vi "IT8512AControl.vi"(8 "功能":T1(ring), 9 "输入":dbl, 10 "端口":string="INP 0") -> (1 "输出":dbl)   [LabVIEW 2018]
uses:
  <vilib>/Instr/_visa.llb/VISA Configure Serial Port (Instr).vi
panel:
  in  "error in (no error)":errorcluster caption="错误输入（无错误）"
  out "error out":errorcluster
  # "IT8512 CONTROL"
  # "r"
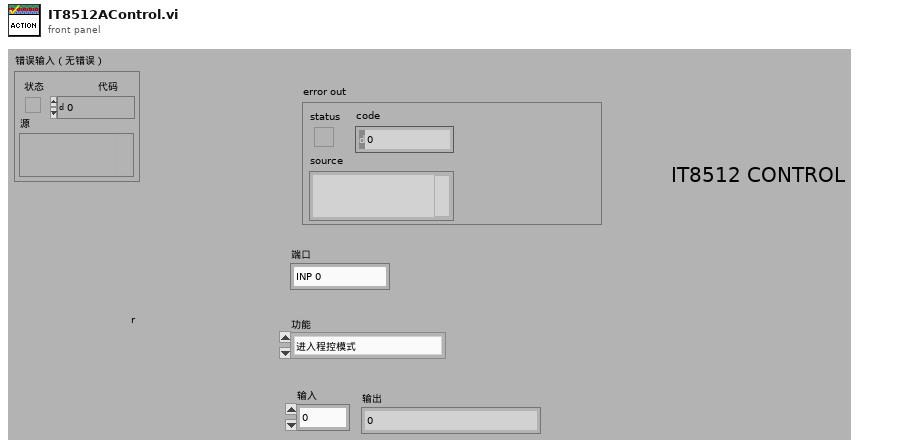
[diagram p1: front panel]
types:
  T1 = enum16{"进入程控模式", "输出ON", "输出OFF", "设置电压", "设置电流", "读取电压", "读取电流", "CC", "CV", "进入手动模式"}
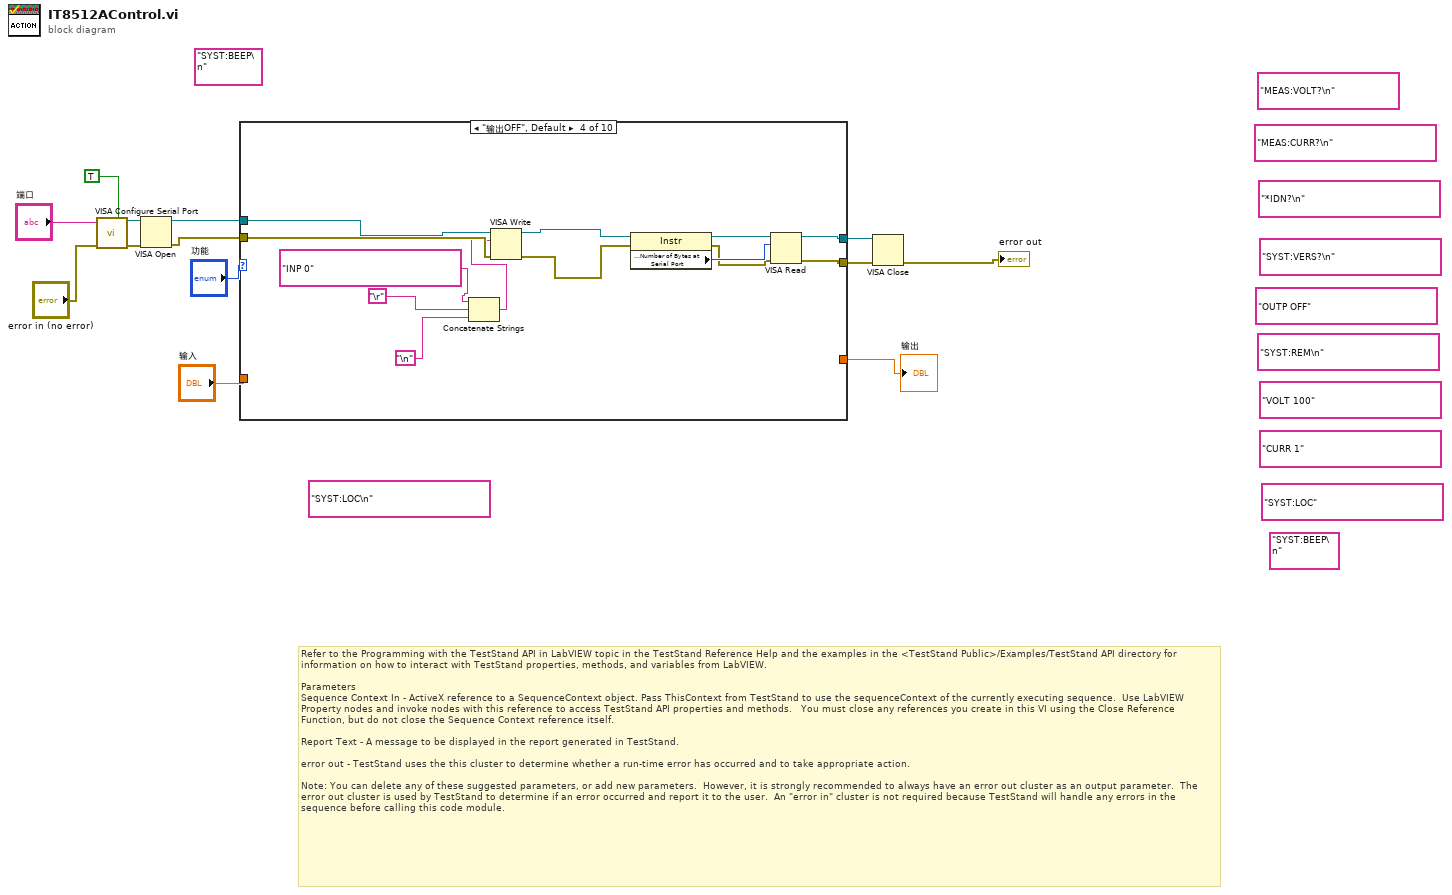
[diagram p0: block diagram]
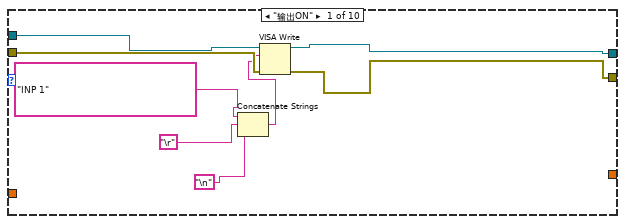
[diagram p2: hidden frame]
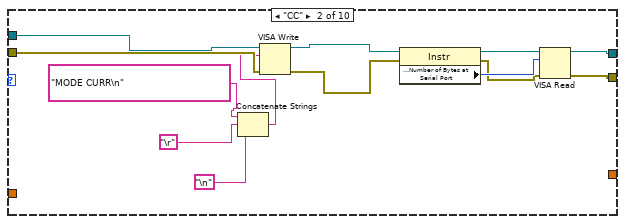
[diagram p3: hidden frame]
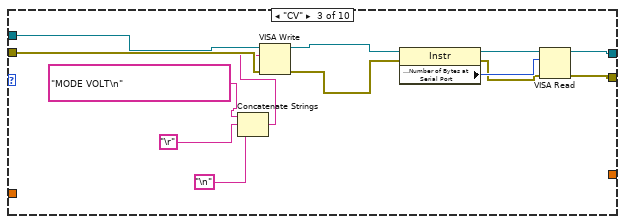
[diagram p4: hidden frame]
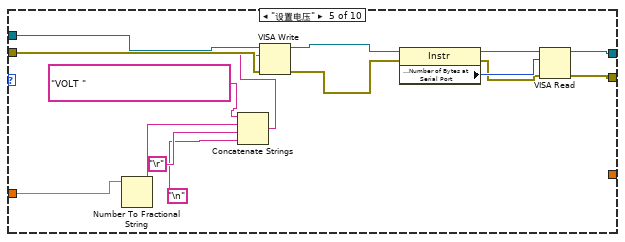
[diagram p5: hidden frame]
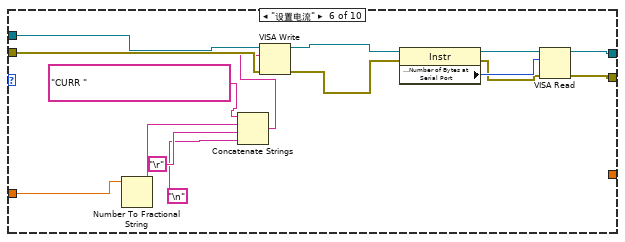
[diagram p6: hidden frame]
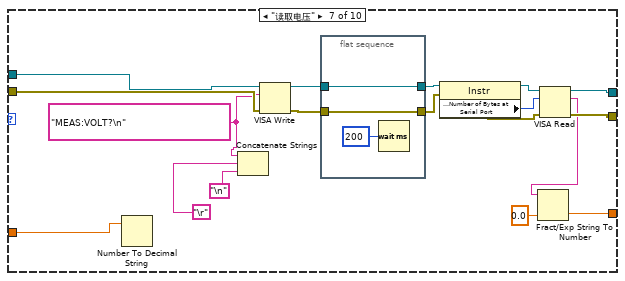
[diagram p7: hidden frame]
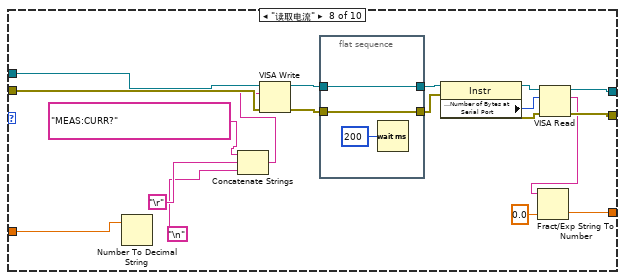
[diagram p8: hidden frame]
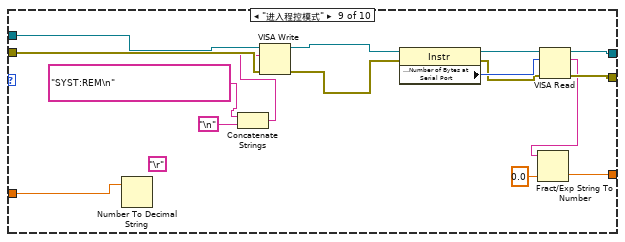
[diagram p9: hidden frame]
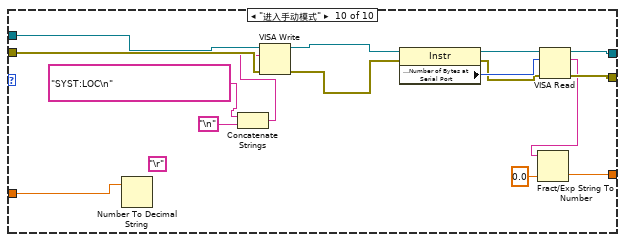
[diagram p10: hidden frame]
diagram:
  (unwired) "SYST:LOC\n" ("写入缓冲区")
  (unwired) "SYST:LOC" ("写入缓冲区")
  (unwired) "CURR 1" ("写入缓冲区")
  (unwired) "VOLT 100" ("写入缓冲区")
  (unwired) "OUTP OFF" ("写入缓冲区")
  (unwired) "SYST:REM\n" ("写入缓冲区")
  (unwired) "SYST:VERS?\n" ("写入缓冲区")
  (unwired) "*IDN?\n" ("写入缓冲区")
  (unwired) "MEAS:CURR?\n" ("写入缓冲区")
  (unwired) "MEAS:VOLT?\n" ("写入缓冲区")
  (unwired) "SYST:BEEP\n" ("写入缓冲区")
  (unwired) "SYST:BEEP\n" ("写入缓冲区")
  # "Refer to the Programming with the TestStand API in LabVIEW topic in the TestStand Reference Help and the examples in the <TestStand Public>/Examples/TestStand API directory for information on how to interact with TestStand properties, methods, and variables from LabVIEW.\n\nParameters\nSequence Context In - ActiveX reference to a SequenceContext object. Pass ThisContext from TestStand to use the sequenceContext of the currently executing sequence.  Use LabVIEW Property nodes and invoke nodes with this reference to access TestStand API properties and methods.   You must close any references you create in this VI using the Close Reference Function, but do not close the Sequence Context reference itself.\n\nReport Text - A message to be displayed in the report generated in TestStand. \n\nerror out - TestStand uses the this cluster to determine whether a run-time error has occurred and to take appropriate action.  \n\nNote: You can delete any of these suggested parameters, or add new parameters.  However, it is strongly recommended to always have an error out cluster as an output parameter.  The error out cluster is used by TestStand to determine if an error occurred and report it to the user.  An \"error in\" cluster is not required because TestStand will handle any errors in the sequence before calling this code module."
  n1 = call-poly "VISA Configure Serial Port"("VISA resource name"="端口", "Enable Termination\nChar (T)"=TRUE ("Enable Termination\nChar (T)"), "error in (no error)"="error in (no error)") -> ("VISA resource name out"=w12:refnum<visa-resource-name>, "error out"=w13:errorcluster)  [unwired: 11 in]
  n2 = VISA Open(error in (no error)=w13, VISA resource name=w12) -> (VISA resource name=w11:refnum<visa-resource-name>, error out=w10:errorcluster)  [unwired: 3 in]
  n3 = case shown="\"输出OFF\", Default" "功能" {
    tunnel: w11 -> [w21 w34 w47 w60 w75 w90 w108 w130 w149 w165]
    tunnel: w10 -> [w20 w33 w46 w59 w74 w89 w107 w129 w148 w164]
    tunnel: [w17 w27 w40 w51 w66 w81 w102 w122 w141 w157] -> w8
    tunnel: [w16 w26 w39 w50 w65 w80 w101 w121 w140 w156] -> w7
    tunnel: "输入" -> [_ _ _ _ w61 w76 w99 w119 w137 w153]
    tunnel: [_ _ _ _ _ _ w96 w116 w134 w150] -> w3
    frame "输出ON" {
      n4 = Concatenate Strings("INP 1" ("写入缓冲区"), "\r", "\n") -> (w14:string)
      n5 = VISA Write(VISA resource name=w21, write buffer=w14, error in (no error)=w20) -> (VISA resource name out=w17:refnum<visa-resource-name>, error out=w16:errorcluster)  [unwired: 1 out]
    }
    frame "CC" {
      n6 = Concatenate Strings("MODE CURR\n" ("写入缓冲区"), "\r", "\n") -> (w28:string)
      n7 = VISA Write(VISA resource name=w34, write buffer=w28, error in (no error)=w33) -> (VISA resource name out=w32:refnum<visa-resource-name>, error out=w24:errorcluster)  [unwired: 1 out]
      n8 = property class="Instr"(reference=w32, error in=w24) -> (reference out=w31:refnum<visa-resource-name>, error out=w25:errorcluster, "Serial Settings:Number of Bytes at Serial Port"=w30:u32)
      n9 = VISA Read(VISA resource name=w31, byte count=w30, error in (no error)=w25) -> (VISA resource name out=w27:refnum<visa-resource-name>, error out=w26:errorcluster)  [unwired: 2 out]
    }
    frame "CV" {
      n10 = Concatenate Strings("MODE VOLT\n" ("写入缓冲区"), "\r", "\n") -> (w41:string)
      n11 = VISA Write(VISA resource name=w47, write buffer=w41, error in (no error)=w46) -> (VISA resource name out=w45:refnum<visa-resource-name>, error out=w37:errorcluster)  [unwired: 1 out]
      n12 = property class="Instr"(reference=w45, error in=w37) -> (reference out=w44:refnum<visa-resource-name>, error out=w38:errorcluster, "Serial Settings:Number of Bytes at Serial Port"=w43:u32)
      n13 = VISA Read(VISA resource name=w44, byte count=w43, error in (no error)=w38) -> (VISA resource name out=w40:refnum<visa-resource-name>, error out=w39:errorcluster)  [unwired: 2 out]
    }
    frame "输出OFF", Default {
      n14 = Concatenate Strings("INP 0" ("写入缓冲区"), "\r", "\n") -> (w54:string)
      n15 = VISA Write(VISA resource name=w60, write buffer=w54, error in (no error)=w59) -> (VISA resource name out=w58:refnum<visa-resource-name>, error out=w48:errorcluster)  [unwired: 1 out]
      n16 = property class="Instr"(reference=w58, error in=w48) -> (reference out=w57:refnum<visa-resource-name>, error out=w49:errorcluster, "Serial Settings:Number of Bytes at Serial Port"=w56:u32)
      n17 = VISA Read(VISA resource name=w57, byte count=w56, error in (no error)=w49) -> (VISA resource name out=w51:refnum<visa-resource-name>, error out=w50:errorcluster)  [unwired: 2 out]
    }
    frame "设置电压" {
      n18 = Number To Fractional String(number=w61) -> (F-format string=w62:string)  [unwired: 3 in]
      n19 = Concatenate Strings("VOLT " ("写入缓冲区"), w62, "\r", "\n") -> (w69:string)
      n20 = VISA Write(VISA resource name=w75, write buffer=w69, error in (no error)=w74) -> (VISA resource name out=w73:refnum<visa-resource-name>, error out=w63:errorcluster)  [unwired: 1 out]
      n21 = property class="Instr"(reference=w73, error in=w63) -> (reference out=w72:refnum<visa-resource-name>, error out=w64:errorcluster, "Serial Settings:Number of Bytes at Serial Port"=w71:u32)
      n22 = VISA Read(VISA resource name=w72, byte count=w71, error in (no error)=w64) -> (VISA resource name out=w66:refnum<visa-resource-name>, error out=w65:errorcluster)  [unwired: 2 out]
    }
    frame "设置电流" {
      n23 = Number To Fractional String(number=w76) -> (F-format string=w77:string)  [unwired: 3 in]
      n24 = Concatenate Strings("CURR " ("写入缓冲区"), w77, "\r", "\n") -> (w84:string)
      n25 = VISA Write(VISA resource name=w90, write buffer=w84, error in (no error)=w89) -> (VISA resource name out=w88:refnum<visa-resource-name>, error out=w78:errorcluster)  [unwired: 1 out]
      n26 = property class="Instr"(reference=w88, error in=w78) -> (reference out=w87:refnum<visa-resource-name>, error out=w79:errorcluster, "Serial Settings:Number of Bytes at Serial Port"=w86:u32)
      n27 = VISA Read(VISA resource name=w87, byte count=w86, error in (no error)=w79) -> (VISA resource name out=w81:refnum<visa-resource-name>, error out=w80:errorcluster)  [unwired: 2 out]
    }
    frame "读取电压" {
      w95 = "MEAS:VOLT?\n" ("写入缓冲区")
      n28 = Number To Decimal String(number=w99) -> ()  [unwired: 1 in, 1 out]
      n29 = Concatenate Strings(w95, "\r", "\n") -> ()  [unwired: 1 out]
      n30 = VISA Write(VISA resource name=w108, write buffer=w95, error in (no error)=w107) -> (VISA resource name out=w93:refnum<visa-resource-name>, error out=w92:errorcluster)  [unwired: 1 out]
      n31 = flat-sequence {
        tunnel: [w111] -> w94
        tunnel: w93 -> [w111]
        tunnel: w92 -> [w110]
        tunnel: [w110] -> w91
        frame #0 {
          n32 = Wait (ms)(milliseconds to wait=u32 200) -> ()  [unwired: 1 out]
        }
      }
      n33 = property class="Instr"(reference=w94, error in=w91) -> (reference out=w106:refnum<visa-resource-name>, error out=w100:errorcluster, "Serial Settings:Number of Bytes at Serial Port"=w105:u32)
      n34 = VISA Read(VISA resource name=w106, byte count=w105, error in (no error)=w100) -> (VISA resource name out=w102:refnum<visa-resource-name>, read buffer=w98:string, error out=w101:errorcluster)  [unwired: 1 out]
      n35 = Fract/Exp String To Number(string=w98, default (0 dbl)=0.0 ("默认(0 I32)")) -> (number=w96:dbl)  [unwired: 2 in, 1 out]
    }
    frame "读取电流" {
      n36 = Number To Decimal String(number=w119) -> ()  [unwired: 1 in, 1 out]
      n37 = Concatenate Strings("MEAS:CURR?" ("写入缓冲区"), "\r", "\n") -> (w125:string)
      n38 = VISA Write(VISA resource name=w130, write buffer=w125, error in (no error)=w129) -> (VISA resource name out=w115:refnum<visa-resource-name>, error out=w114:errorcluster)  [unwired: 1 out]
      n39 = flat-sequence {
        tunnel: [w133] -> w113
        tunnel: w115 -> [w133]
        tunnel: w114 -> [w132]
        tunnel: [w132] -> w112
        frame #0 {
          n40 = Wait (ms)(milliseconds to wait=u32 200) -> ()  [unwired: 1 out]
        }
      }
      n41 = property class="Instr"(reference=w113, error in=w112) -> (reference out=w128:refnum<visa-resource-name>, error out=w120:errorcluster, "Serial Settings:Number of Bytes at Serial Port"=w127:u32)
      n42 = VISA Read(VISA resource name=w128, byte count=w127, error in (no error)=w120) -> (VISA resource name out=w122:refnum<visa-resource-name>, read buffer=w118:string, error out=w121:errorcluster)  [unwired: 1 out]
      n43 = Fract/Exp String To Number(string=w118, default (0 dbl)=0.0 ("默认(0 I32)")) -> (number=w116:dbl)  [unwired: 2 in, 1 out]
    }
    frame "进入程控模式" {
      (unwired) "\r"
      n44 = Number To Decimal String(number=w137) -> ()  [unwired: 1 in, 1 out]
      n45 = Concatenate Strings("SYST:REM\n" ("写入缓冲区"), "\n") -> (w143:string)
      n46 = VISA Write(VISA resource name=w149, write buffer=w143, error in (no error)=w148) -> (VISA resource name out=w147:refnum<visa-resource-name>, error out=w138:errorcluster)  [unwired: 1 out]
      n47 = property class="Instr"(reference=w147, error in=w138) -> (reference out=w146:refnum<visa-resource-name>, error out=w139:errorcluster, "Serial Settings:Number of Bytes at Serial Port"=w145:u32)
      n48 = VISA Read(VISA resource name=w146, byte count=w145, error in (no error)=w139) -> (VISA resource name out=w141:refnum<visa-resource-name>, read buffer=w136:string, error out=w140:errorcluster)  [unwired: 1 out]
      n49 = Fract/Exp String To Number(string=w136, default (0 dbl)=0.0 ("默认(0 I32)")) -> (number=w134:dbl)  [unwired: 2 in, 1 out]
    }
    frame "进入手动模式" {
      (unwired) "\r"
      n50 = Number To Decimal String(number=w153) -> ()  [unwired: 1 in, 1 out]
      n51 = Concatenate Strings("SYST:LOC\n" ("写入缓冲区"), "\n") -> (w159:string)
      n52 = VISA Write(VISA resource name=w165, write buffer=w159, error in (no error)=w164) -> (VISA resource name out=w163:refnum<visa-resource-name>, error out=w154:errorcluster)  [unwired: 1 out]
      n53 = property class="Instr"(reference=w163, error in=w154) -> (reference out=w162:refnum<visa-resource-name>, error out=w155:errorcluster, "Serial Settings:Number of Bytes at Serial Port"=w161:u32)
      n54 = VISA Read(VISA resource name=w162, byte count=w161, error in (no error)=w155) -> (VISA resource name out=w157:refnum<visa-resource-name>, read buffer=w152:string, error out=w156:errorcluster)  [unwired: 1 out]
      n55 = Fract/Exp String To Number(string=w152, default (0 dbl)=0.0 ("默认(0 I32)")) -> (number=w150:dbl)  [unwired: 2 in, 1 out]
    }
  }
  "输出" <- w3
  n56 = VISA Close(VISA resource name=w8, error in (no error)=w7) -> (error out=→"error out":errorcluster)
